vi "Count Pixels.vi"(3 "Error":string, 4 "Pixel Value":u8, 5 "Input Image 1":T1={"Image ID"=0, "Channel ID"=-1}) -> (0 "Error":string, 1 "Count":u32, 2 "Input Image 1":T1={"Image ID"=0, "Channel ID"=-1})   [LabVIEW 2011, in "labvvis.lvlib"]
doc: "Adds each pixel from Input Image 1 with the corresponding pixel from Input Image 2. The result is written to Output Image. If the result is greater than 255, then the result is 255."
uses:
  <userlib>/labvvis/labvvis.lvlib
  <userlib>/labvvis/VVIS Image.ctl
  labvvis.framework
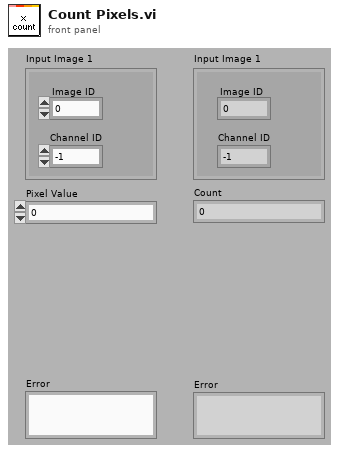
[diagram p1: front panel]
types:
  T1 = typedef "labvvis.lvlib/VVIS Image.ctl" = cluster{"Image ID":i16, "Channel ID":i16}
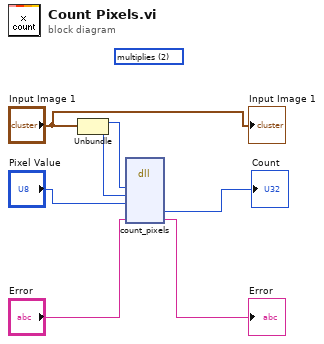
[diagram p0: block diagram]
diagram:
  (unwired) u8 2 items=["plus_saturated", "minus_saturated", "multiplies", "divides", "modulus", "equal_to", "not_equal_to", "greater", "greater_equal", "less", "less_equal", "logical_and", "logical_or", "bitwise_and", "bitwise_or"] ("Function")
  n1 = Unbundle("Input Image 1") -> ("Image ID"=w6:i16, "Channel ID"=w5:i16)
  n2 = dll-call lib="labvvis.framework" fn="count_pixels"("src1"=w6, "cid1"=w5, "pixel"="Pixel Value", "error"="Error") -> ("count"=→"Count":u32, "error"=→"Error":string)  [unwired: 8 in, 2 out]
  "Input Image 1" <- "Input Image 1"
